vi "Double to Number 2dp units below.vi"(4 "Unit":string, 8 "Number":dbl) -> (3 "Number string":string)   [LabVIEW 2014]
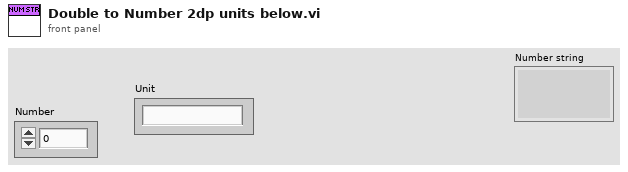
[diagram p1: front panel]
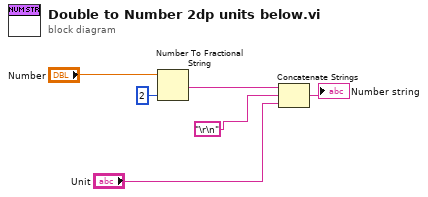
[diagram p0: block diagram]
diagram:
  n1 = Number To Fractional String(number="Number", precision (6)=i16 2) -> (F-format string=w4:string)  [unwired: 2 in]
  n2 = Concatenate Strings(w4, "\r\n", "Unit") -> (→"Number string":string)
